vi "crio_FPGA_Load_Cell.vi"() -> ()   [LabVIEW 2019]
uses:
  <vilib>/rvi/Emulation/niFpgaSctlEmulationGetInTimedLoop.vi
  <vilib>/rvi/Emulation/niFpgaProcessEmulError.vi
  <vilib>/rvi/Emulation/niFpgaGetClockAttributes.vi
  <vilib>/rvi/Emulation/niFpgaEmulationReportErrorSimple.vi
  <vilib>/rvi/eio/common/nirviEmuTemplateMethod_errors.vi
  <vilib>/rvi/Emulation/niFpgaCriticalErrorInLSC.vi
  <vilib>/eio/EIONode/EIONode.xnode
panel:
  out "Difference AI2 AI3":fxp<+/-,27,6>
  out "Mod5/AI3":fxp<+/-,26,5>
  out "Mod5/AI2":fxp<+/-,26,5>
  out "Difference":fxp<+/-,27,6>
  out "Mod5/AI1":fxp<+/-,26,5>
  in  "stop":bool
  out "Mod5/AI0":fxp<+/-,26,5>
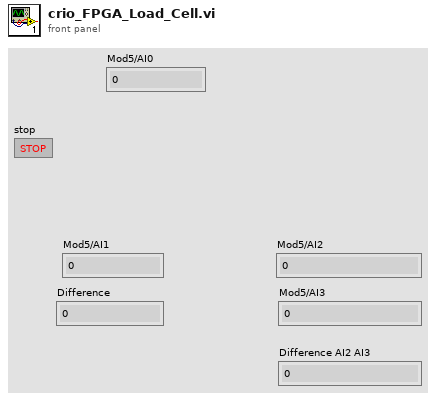
[diagram p1: front panel]
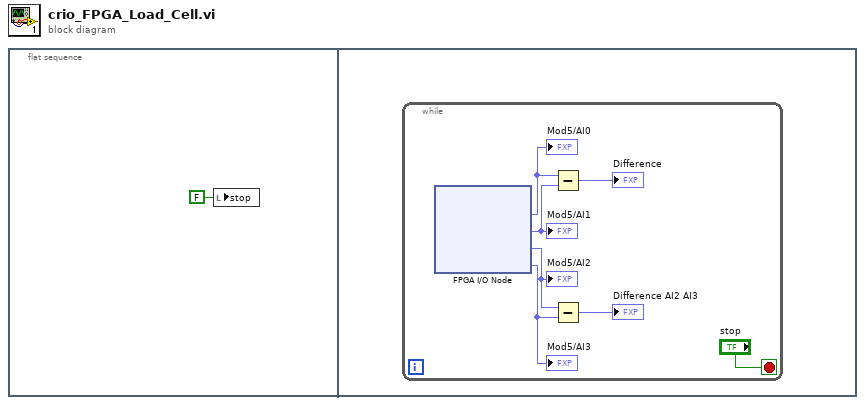
[diagram p0: block diagram]
diagram:
  n1 = flat-sequence {
    frame #0 {
      n2 = local write "stop"(FALSE ("stop")) -> ()
    }
    frame #1 {
      n3 = while {
        stop <- "stop" stop-if-true
        n4 = xnode "FPGA I/O Node"() -> ("Mod5/AI0"=w7:fxp<+/-,26,5>, "Mod5/AI1"=w6:fxp<+/-,26,5>, "Mod5/AI2"=w4:fxp<+/-,26,5>, "Mod5/AI3"=w3:fxp<+/-,26,5>)  [unwired: 4 in, 4 out]
        "Mod5/AI0" <- w7
        "Mod5/AI1" <- w6
        "Mod5/AI2" <- w4
        "Mod5/AI3" <- w3
        n5 = Subtract(x=w7, y=w6) -> (x-y=→"Difference":fxp<+/-,27,6>)
        n6 = Subtract(x=w4, y=w3) -> (x-y=→"Difference AI2 AI3":fxp<+/-,27,6>)
      }
    }
  }
